vi "Terminal-Core-UDPModule.vi"(8 "error in":errorcluster, 9 "ErrorQRef":refnum<queue>, 10 "DataQRef":refnum<queue>, 11 "UdpQRef":refnum<queue>) -> (0 "错误输出":errorcluster)   [LabVIEW 2014]
panel:
  out "x+1":i32
  in  "开关":bool=TRUE
  out "Udp::Initialize":string
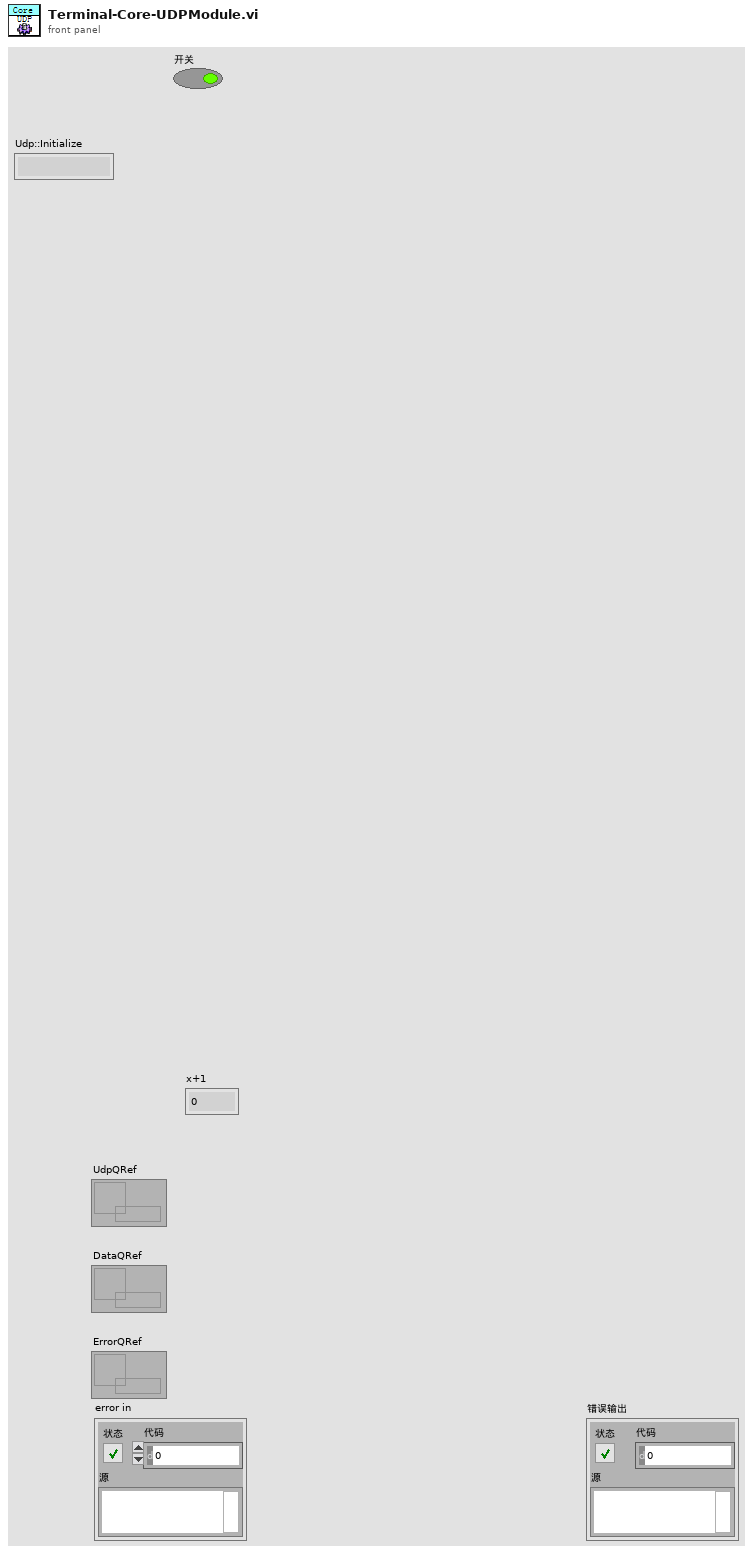
[diagram p1: front panel]
types:
  T1 = cluster{"设备名":string, "时间":timestamp, "数据":sgl[][], "通道长度":i32[], "次数":i32}
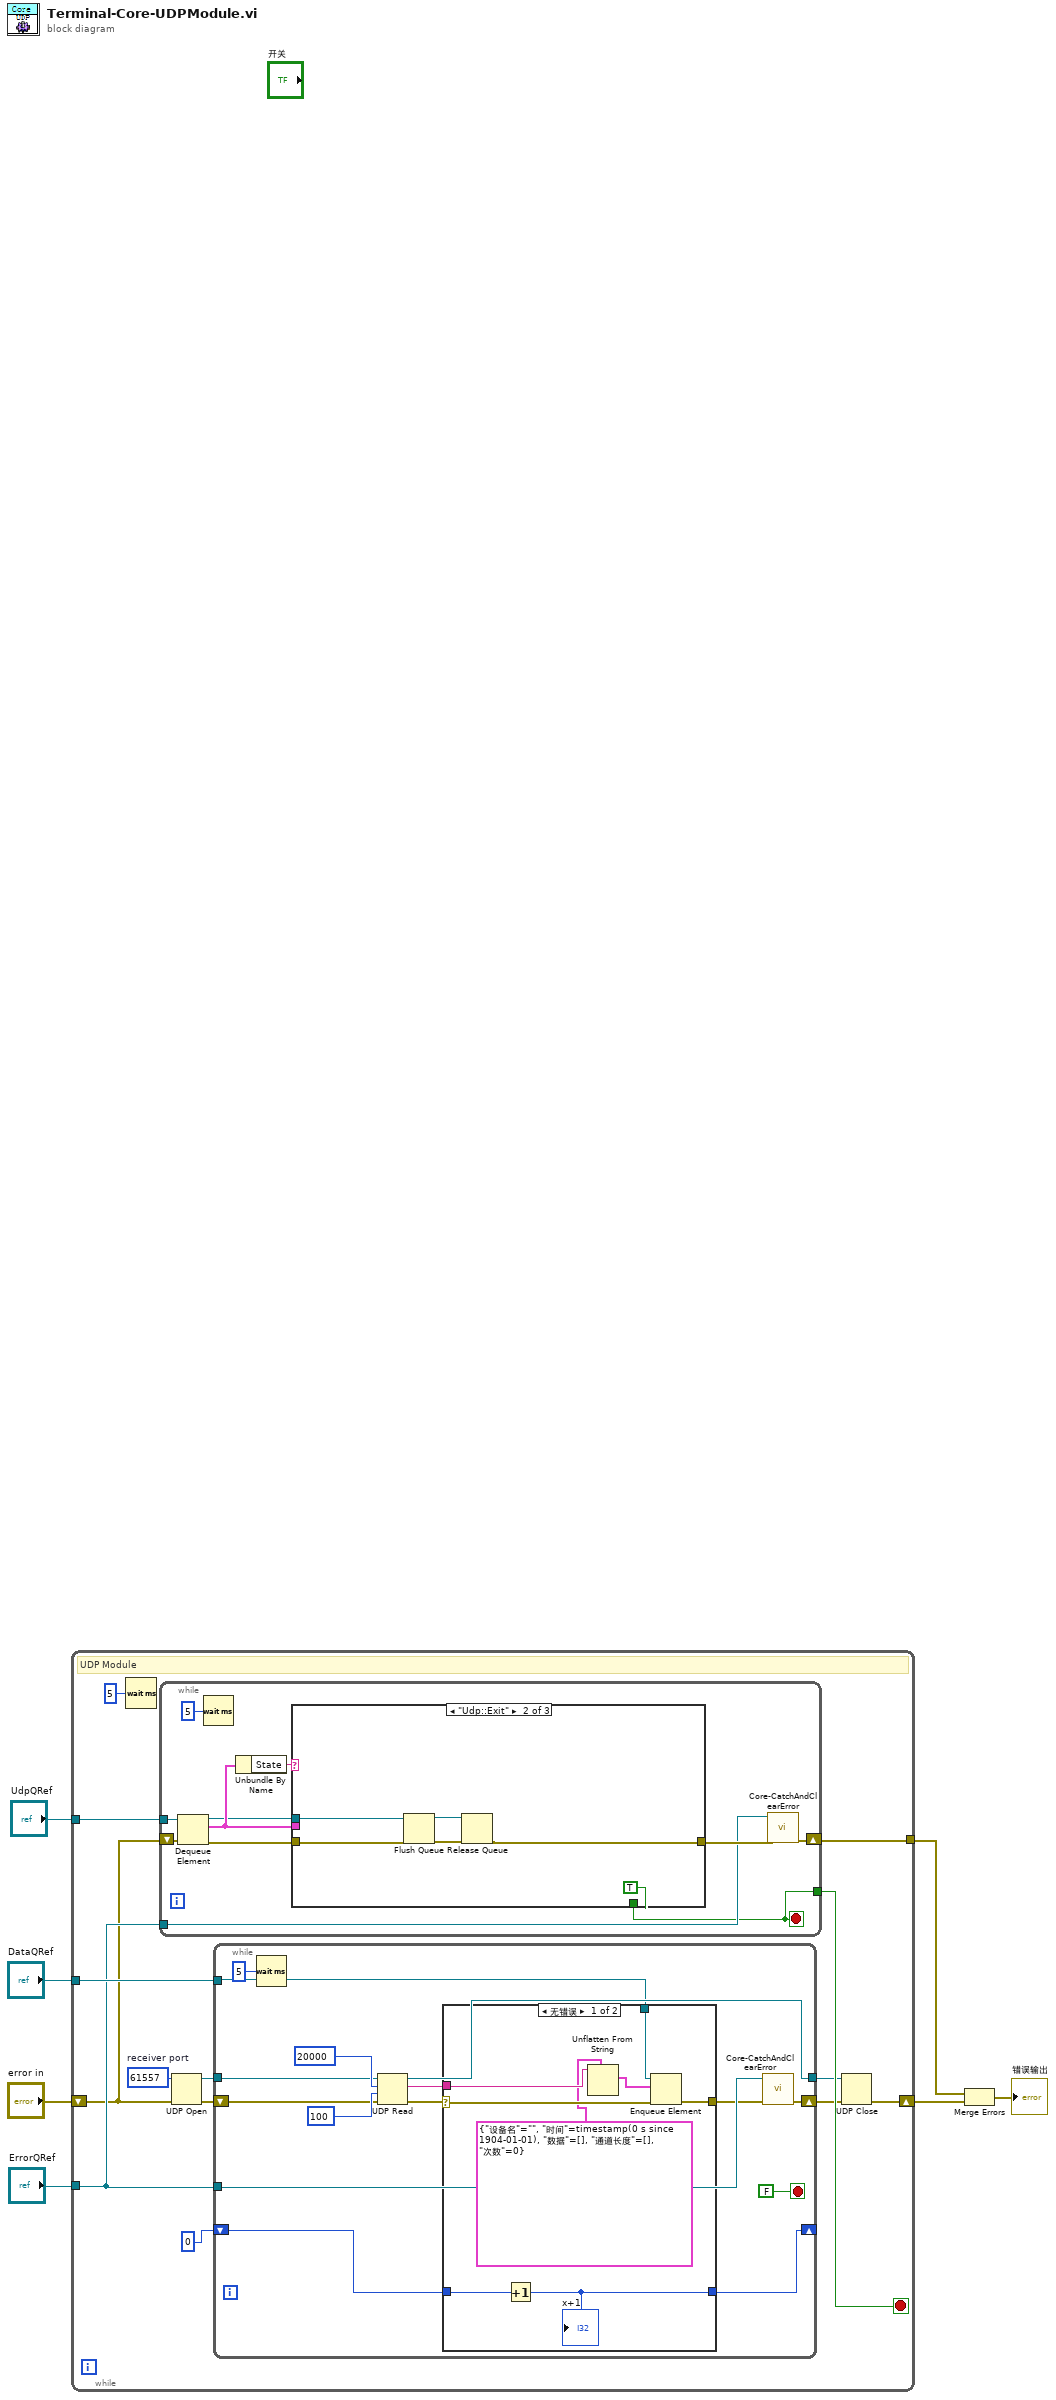
[diagram p0: block diagram]
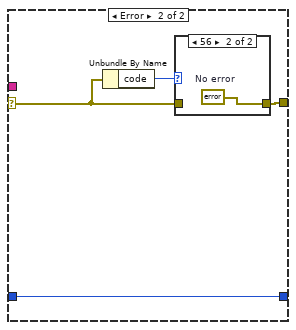
[diagram p2: hidden frame]
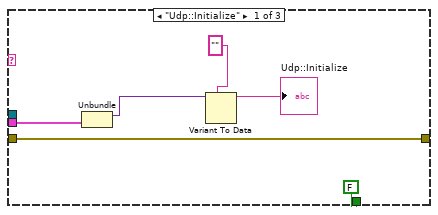
[diagram p4: hidden frame]
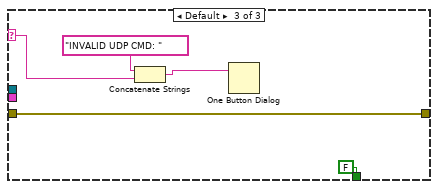
[diagram p5: hidden frame]
diagram:
  n1 = while {
    tunnel: "DataQRef" -> [w19]
    shift-right: [w14] -> w5
    shift-left: "error in" -> [w15]
    tunnel: "ErrorQRef" -> [w17]
    tunnel: "UdpQRef" -> [w20]
    tunnel: [w16] -> w4
    stop <- w18 stop-if-true
    w13 = u16 61557  # receiver port
    # "UDP Module"
    n2 = Wait (ms)(milliseconds to wait=u32 5 ("等待时间（毫秒）")) -> ()  [unwired: 1 out]
    n3 = while {
      tunnel: w20 -> [w61]
      tunnel: [w52] -> w18
      tunnel: w17 -> [w53]
      shift-right: [w59] -> w16
      shift-left: w15 -> [w60]
      stop <- w52 stop-if-true
      n4 = Dequeue Element(queue=w61, error in (no error)=w60) -> (queue out=w54:refnum<queue>, element=w58:cluster{"Data":variant, "State":string}, error out=w56:errorcluster)  [unwired: 1 in, 1 out]
      n5 = Wait (ms)(milliseconds to wait=u32 5 ("等待时间（毫秒）")) -> ()  [unwired: 1 out]
      n6 = Unbundle By Name(w58) -> ("State"=w57:string)
      n7 = case shown="\"Udp::Exit\"" w57 {
        selector: w57 -> [_ _ w76]
        tunnel: w58 -> [w65 _ _]
        tunnel: w56 -> [w67 w71 w75]
        tunnel: [w67 w70 w75] -> w55
        tunnel: w54 -> [_ w69 _]
        tunnel: [FALSE TRUE FALSE] -> w52
        frame "Udp::Initialize" {
          n8 = Unbundle(w65) -> ("Data"=w66:variant)  [unwired: 1 out]
          n9 = Variant To Data(type="", Variant=w66) -> (data=→"Udp::Initialize":string)  [unwired: 1 in, 1 out]
        }
        frame "Udp::Exit" {
          n10 = Flush Queue(queue=w69, error in (no error)=w71) -> (queue out=w73:refnum<queue>, error out=w72:errorcluster)  [unwired: 1 out]
          n11 = Release Queue(queue=w73, error in (no error)=w72) -> (error out=w70:errorcluster)  [unwired: 1 in, 2 out]
        }
        frame Default {
          n12 = Concatenate Strings("INVALID UDP CMD: ", w76) -> (w77:string)
          n13 = One Button Dialog(message=w77) -> ()  [unwired: 1 in, 1 out]
        }
      }
      n14 = call "Core-CatchAndClearError.vi"("error in (no error)"=w55, "ErrorQ"=w53) -> ("error out"=w59:errorcluster)  [unwired: 7 in]
    }
    n15 = UDP Open(8:w15, 11:w13) -> (port=w12:refnum<k16>, 0:w11:errorcluster)  [unwired: 3 in, 1 out]
    n16 = while {
      tunnel: w17 -> [w29]
      tunnel: w19 -> [w25]
      tunnel: w12 -> [w33]
      shift-right: [w30] -> w10
      shift-left: w11 -> [w32]
      tunnel: [w27] -> w9
      shift-right: [w22] -> _
      shift-left: 0 -> [w23]
      stop <- FALSE stop-if-true
      n17 = Wait (ms)(milliseconds to wait=u32 5 ("等待时间（毫秒）")) -> ()  [unwired: 1 out]
      n18 = UDP Read(connection ID=w33, max size (548)=20000 ("最大值(548)"), timeout ms (25000)=100, 8:w32) -> (data out=w26:string, error out=w28:errorcluster, 3:w27:refnum<k16>)  [unwired: 2 out]
      n19 = case shown="无错误" w28 {
        selector: w28 -> [w43 w46]
        tunnel: w26 -> [w41 _]
        tunnel: w25 -> [w44 _]
        tunnel: [w42 w47] -> w24
        tunnel: w23 -> [w38 w45]
        tunnel: [w37 w45] -> w22
        frame No Error {
          n20 = Increment(x=w38) -> (x+1=w37:i32)
          "x+1" <- w37
          n21 = Unflatten From String(type=T1 {"设备名"="", "时间"=timestamp(0 s since 1904-01-01), "数据"=[], "通道长度"=[], "次数"=0}, binary string=w41) -> (value=w40:T1)  [unwired: 3 in, 2 out]
          n22 = Enqueue Element(queue=w44, element=w40, error in (no error)=w43) -> (error out=w42:errorcluster)  [unwired: 1 in, 2 out]
        }
        frame Error {
          n23 = Unbundle By Name(w46) -> ("code"=w48:i32)
          n24 = case shown="56" w48 {
            tunnel: w46 -> [w49 _]
            tunnel: [w49 w50] -> w47
            frame Default {
            }
            frame 56 {
              w50 = errorcluster {"status"=FALSE, "code"=0, "source"=""}  # No error
            }
          }
        }
      }
      n25 = call "Core-CatchAndClearError.vi"("error in (no error)"=w24, "ErrorQ"=w29) -> ("error out"=w30:errorcluster)  [unwired: 7 in]
    }
    n26 = UDP Close(connection ID=w9, 8:w10) -> (error out=w14:errorcluster)  [unwired: 1 out]
  }
  n27 = Merge Errors(w4, w5) -> (→"错误输出":errorcluster)
